vi "Close GUI.vi"(8 "error in":errorcluster, 11 "Main GUI VI Reference In":refnum<vi>) -> (0 "error out":errorcluster, 3 "Main GUI VI Reference Out":refnum<vi>)   [LabVIEW 2017, in "DTacq Plot Display Library.lvlib"]
doc: "Close the graphical user interface"
uses:
  DTacq Plot Display Library.lvlib
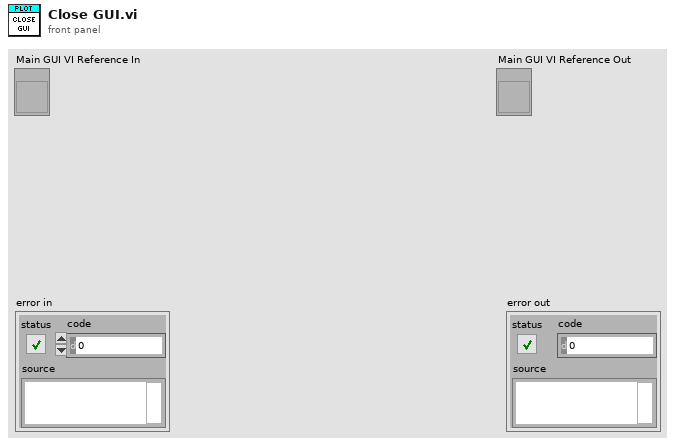
[diagram p1: front panel]
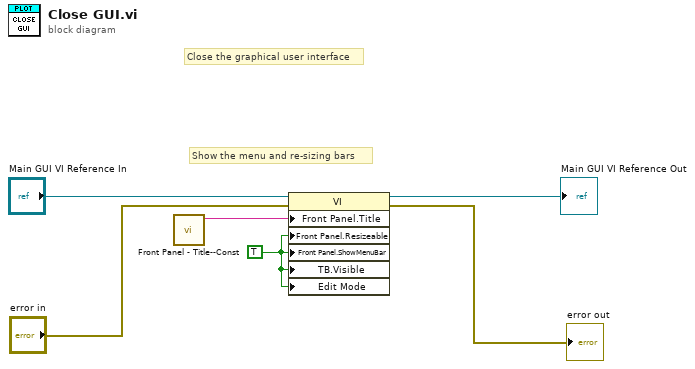
[diagram p0: block diagram]
diagram:
  w1 = TRUE ("Front Panel Window:Show Menu Bar")
  # "Show the menu and re-sizing bars"
  # "Close the graphical user interface"
  n1 = call "Front Panel - Title--Const.vi"() -> ("Window Title"=w3:string)  [unwired: 11 in]
  n2 = property class="VI"(reference="Main GUI VI Reference In", error in="error in", "Front Panel.Title"=w3, "Front Panel.Resizeable"=w1, "Front Panel.ShowMenuBar"=w1, "TB.Visible"=w1, "Edit Mode"=w1) -> (reference out=→"Main GUI VI Reference Out":refnum<vi>, error out=→"error out":errorcluster)
